vi "Is Critical Alarm Set.vi"(11 "alarms":T1(array[cluster])) -> (3 "critical alarm?":bool)   [LabVIEW 2018, in "Dynamic Shared Variables.lvlib"]
doc: "Takes the raw Alarm events and creates an Alarm Model and the display to show the alarm ribbon bar."
uses:
  Dynamic Shared Variables.lvlib
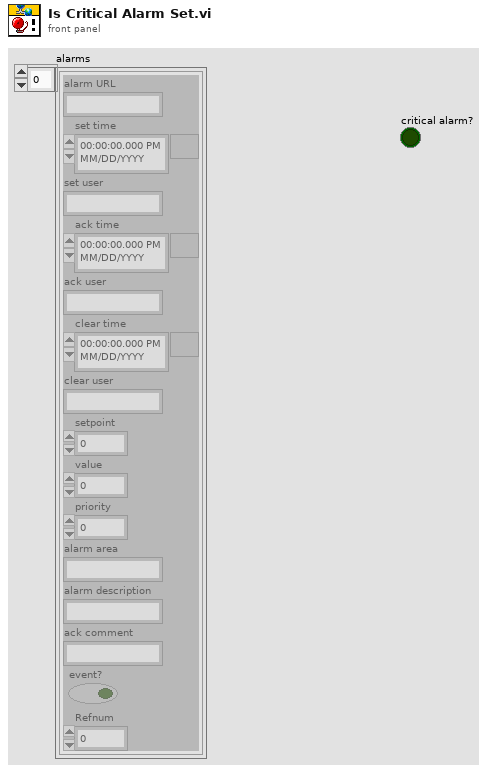
[diagram p1: front panel]
types:
  T1 = cluster{"alarm URL":string, "set time":timestamp, "set user":string, "ack time":timestamp, "ack user":string, "clear time":timestamp, "clear user":string, "setpoint":dbl, "value":dbl, "priority":u32, "alarm area":string, "alarm description":string, "ack comment":string, "event?":bool, "Refnum":u64}[]
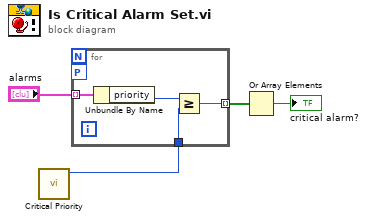
[diagram p0: block diagram]
diagram:
  n1 = call "Critical Priority.vi"() -> ("critical priority"=w3:i32)  [unwired: 11 in]
  n2 = for {
    tunnel: "alarms" -> [w8] mode=indexing
    tunnel: w3 -> [w6]
    tunnel: [w5] -> w2 mode=indexing
    workers-P: _ -> [_]
    n3 = Unbundle By Name(w8) -> ("priority"=w7:u32)
    n4 = Greater Or Equal?(x=w7, y=w6) -> (x >= y?=w5:bool)
  }
  n5 = Or Array Elements(Boolean array=w2) -> (logical OR=→"critical alarm?":bool)
